vi "4.6.1.vi"() -> ()   [LabVIEW 2017]
panel:
  in  "stop":bool
  out "和":dbl
  in  "b":dbl
  in  "a":dbl
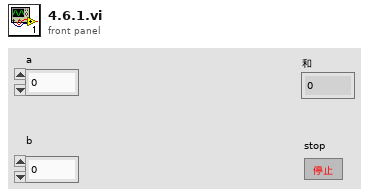
[diagram p1: front panel]
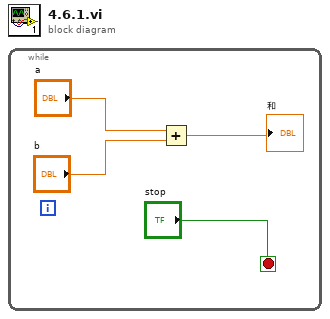
[diagram p0: block diagram]
diagram:
  n1 = while {
    stop <- "stop" stop-if-true
    n2 = Add(x="a", y="b") -> (x+y=→"和":dbl)
  }
